vi "GetLocalReference.vi"(8 "error in":errorcluster, 11 "Local in":refnum<class "Local.lvclass">) -> (0 "error out":errorcluster, 1 "reference out":refnum<vi>, 3 "Local out":refnum<class "Local.lvclass">)   [LabVIEW 2014, in "Local.lvclass"]
uses:
  Local.lvclass
  Generic/Generic.lvclass
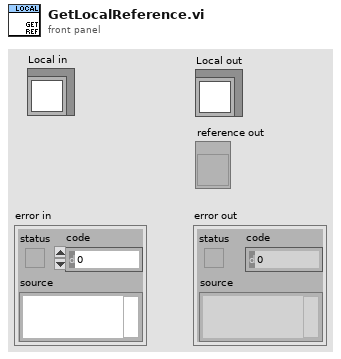
[diagram p1: front panel]
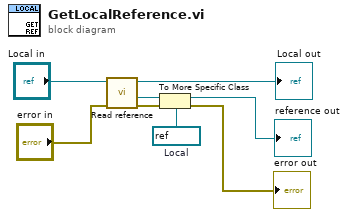
[diagram p0: block diagram]
diagram:
  w5 = refnum<vi> refnum  # Local
  n1 = call "Read reference.vi"("error in"="error in", "GObject in"="Local in") -> ("error out"=w6:errorcluster, "reference"=w7:refnum<vi>, "GObject out"=→"Local out":refnum<class "Local.lvclass">)  [unwired: 5 in]
  n2 = To More Specific Class(target class=w5, reference=w7, error in=w6) -> (specific class reference=→"reference out":refnum<vi>, error out=→"error out":errorcluster)
